vi "OAT Convert Phase.vi"   [LabVIEW 2017]
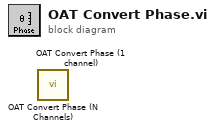
[diagram p0: block diagram]
diagram:
  n1 = call <vilib>:"OAT Convert Phase (N Channels).vi"() -> ()  [unwired: 11 in, 1 out]
  n2 = call <vilib>:"OAT Convert Phase (1 channel).vi"() -> ()  [unwired: 11 in, 1 out]
